vi "main.vi"() -> ()   [LabVIEW 2018]
uses:
  gbl.vi
panel:
  out "保存组数":i32
  in  "保存开关":bool
  out "监测组数":i32
  in  "监测开关":bool
  in  "采样开关":bool
  in  "报警窗":i32(listbox)
  in  "闸门四高度":i32(slide) caption="高  度" scale=0.0..50.0
  in  "闸门四宽度":i32(slide) caption="宽  度" scale=0.0..10.0
  in  "闸门四起点":i32(slide) caption="起  点" scale=0.0..10.0
  in  "闸门三高度":i32(slide) caption="高  度" scale=0.0..50.0
  in  "闸门三宽度":i32(slide) caption="宽  度" scale=0.0..10.0
  in  "闸门三起点":i32(slide) caption="起  点" scale=0.0..10.0
  in  "闸门二高度":i32(slide) caption="高  度" scale=0.0..50.0
  in  "闸门二宽度":i32(slide) caption="宽  度" scale=0.0..10.0
  in  "闸门二起点":i32(slide) caption="起  点" scale=0.0..10.0
  in  "闸门一高度":i32(slide) caption="高  度" scale=0.0..50.0
  in  "闸门一宽度":i32(slide) caption="宽  度" scale=0.0..10.0
  in  "闸门一起点":i32(slide) caption="起  点" scale=0.0..10.0
  in  "衰减上限":dbl
  in  "衰减实时值":dbl
  out "衰  减":bool
  in  "数据导出路径":string
  in  "衰减下限":dbl
  in  "声速上限":dbl
  in  "声速实时值":dbl
  out "声  速":bool
  out "连接状态":bool
  in  "本次监测名称":string
  out "实时信号":cluster{"波形数据":dbl[], "波形数据":dbl[]}[](graph)
  in  "声速下限":dbl
  in  "测    试":bool
  in  "监    测":bool
  in  "采    样":bool
  out "实时监测":cluster{"Value":timestamp[], "Value":dbl[]}[](graph)
  # "声速"
  # "衰减"
  # "时间"
  # "时间"
  # "上    限"
  # "实时值"
  # "下    限"
  # "原 始 信 号"
  # "幅值"
  # "闸  门  一"
  # "闸  门  二"
  # "闸  门  三"
  # "闸  门  四"
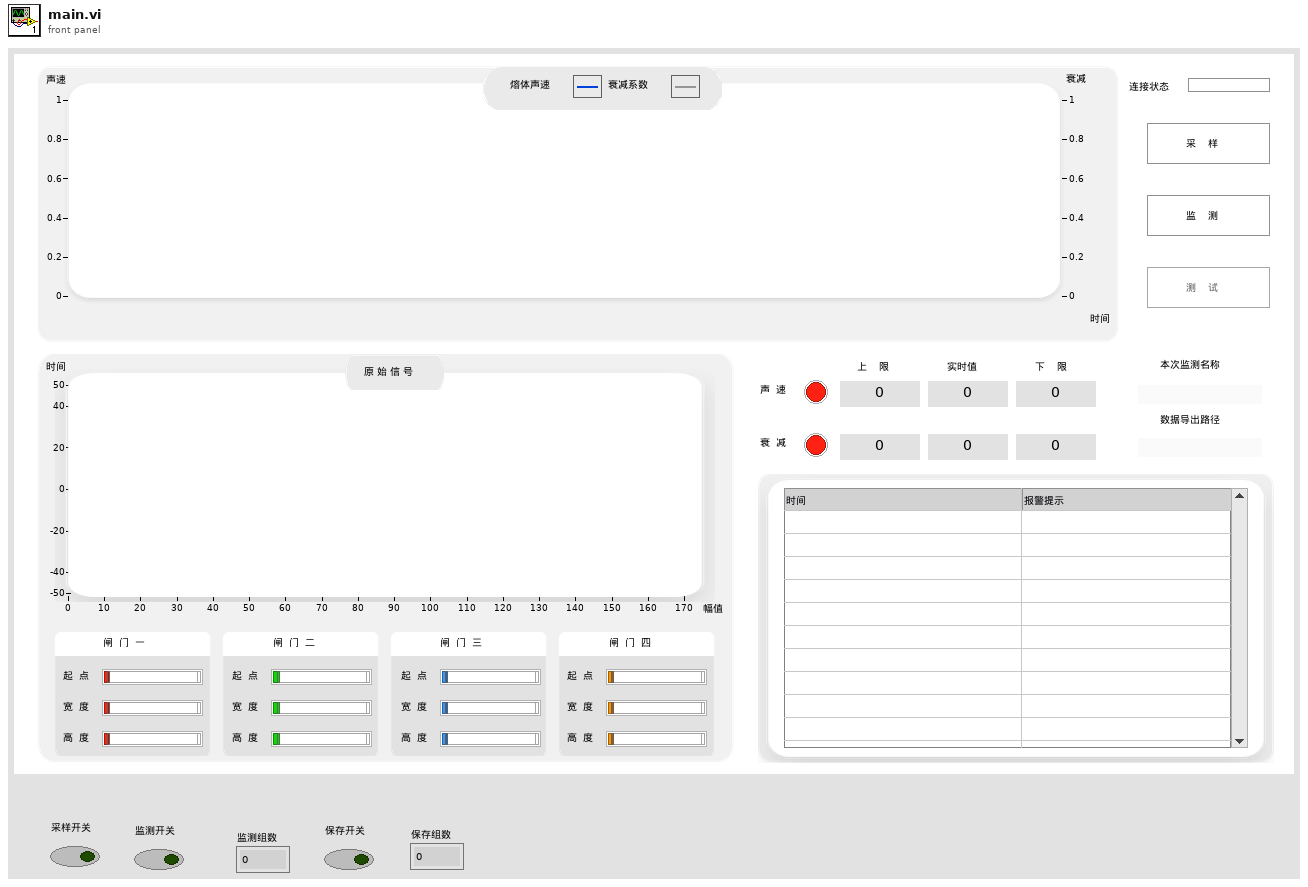
[diagram p1: front panel]
types:
  T1 = enum8{"Enabled", "Disabled", "Disabled and Grayed Out"}
  T2 = enum32{"Bad", "Idle", "Run top level", "Running"}
  T3 = enum32{"Invalid", "Standard", "Closed", "Hidden", "Minimized", "Maximized"}
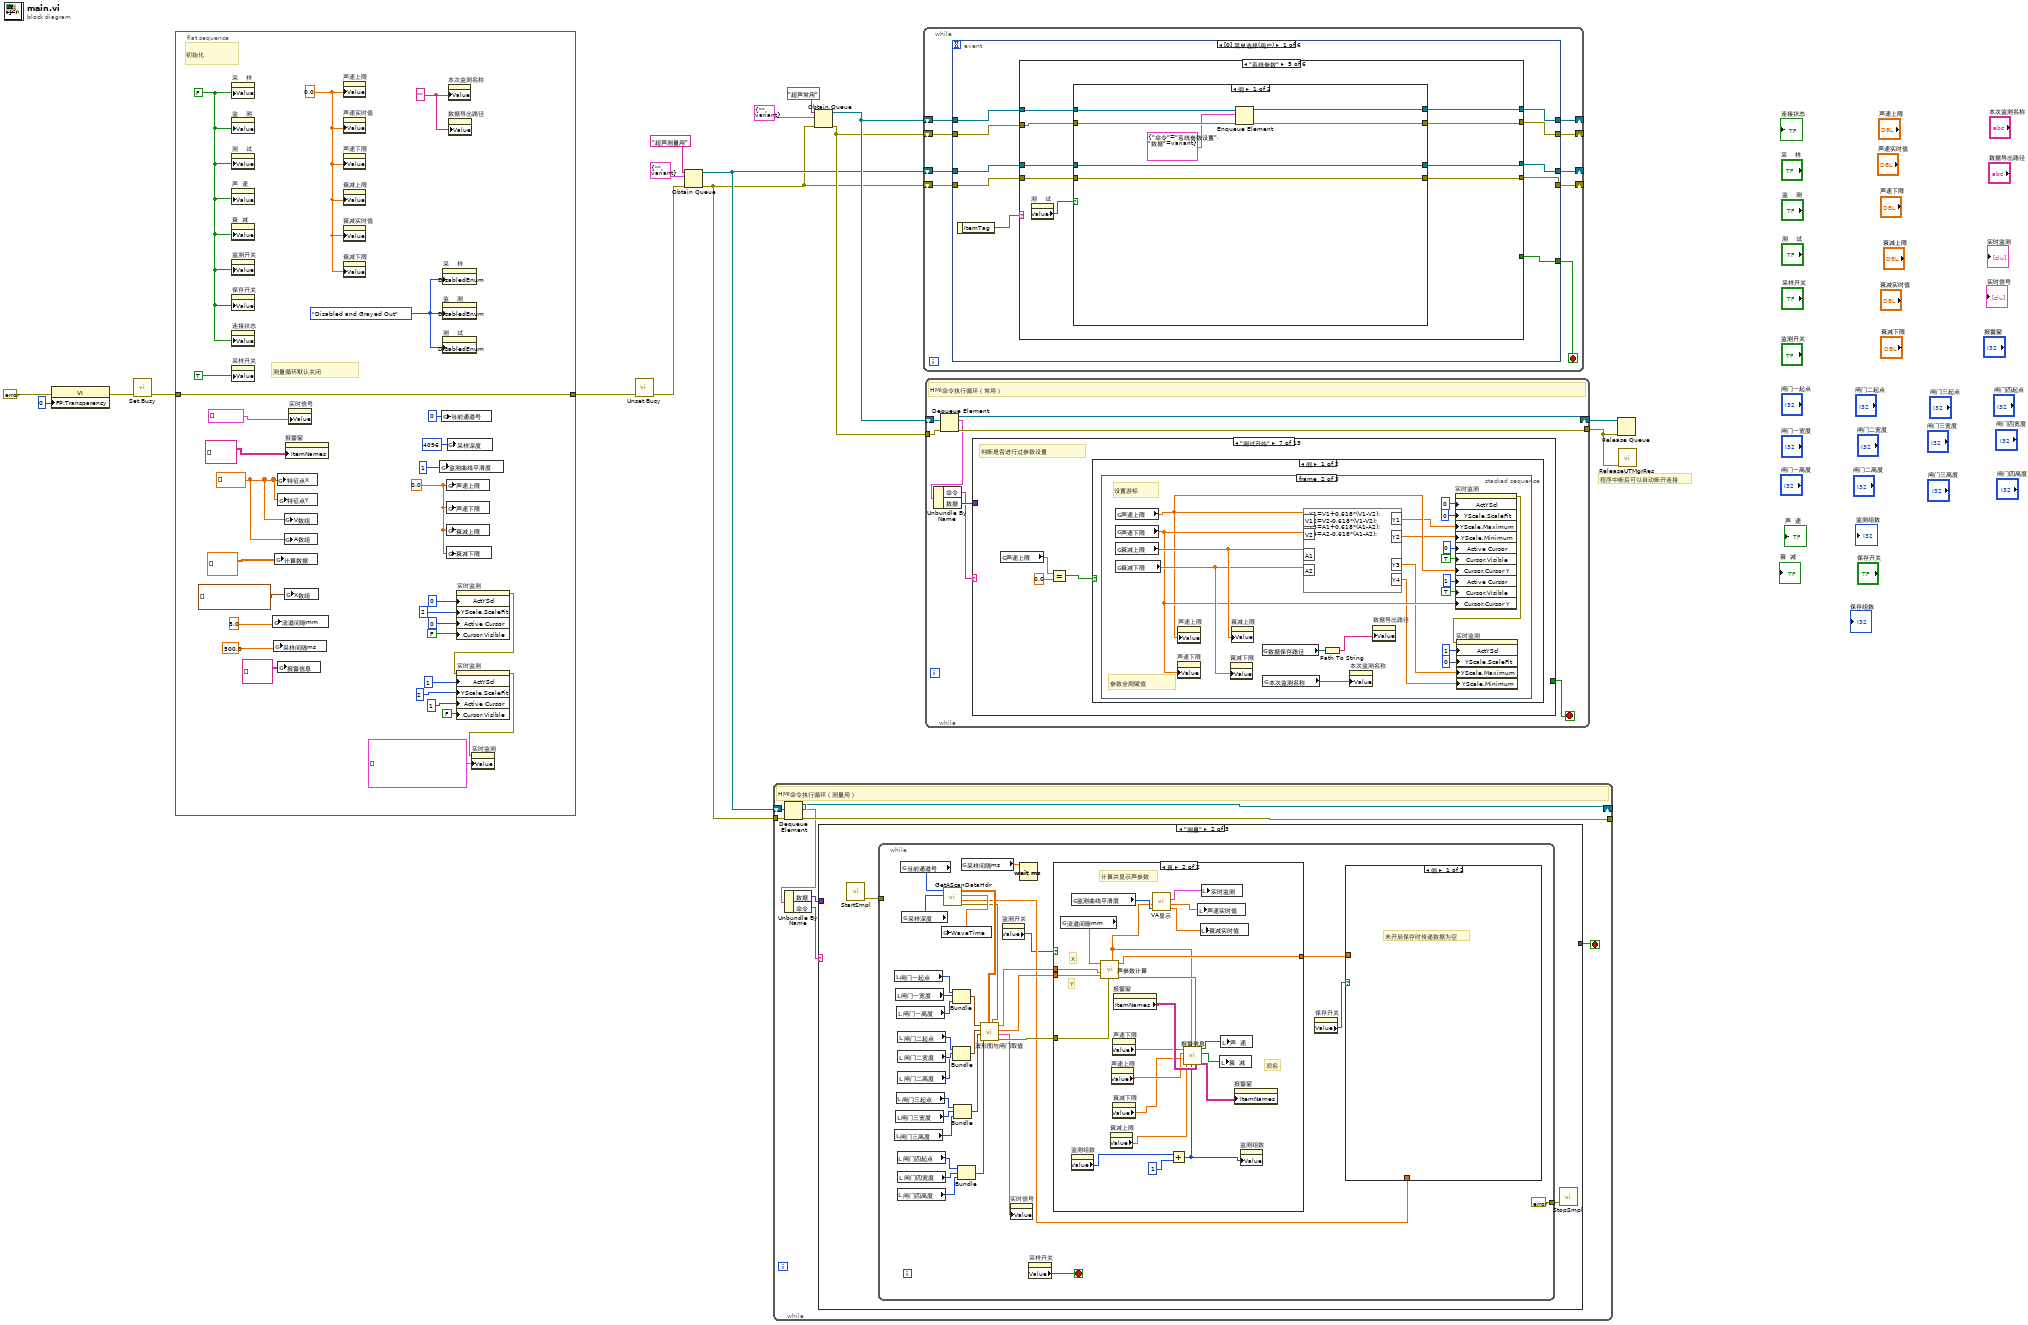
[diagram p0: block diagram]
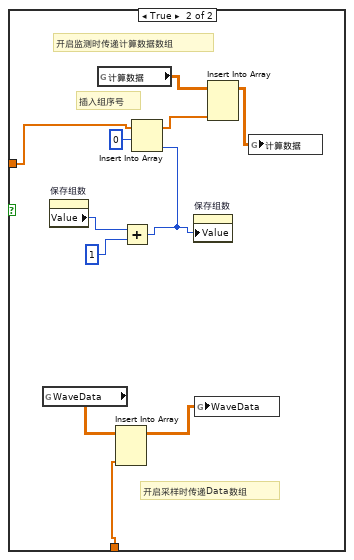
[diagram p3: hidden frame]
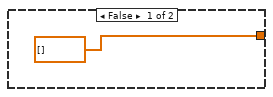
[diagram p4: hidden frame]
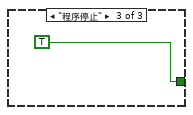
[diagram p5: hidden frame]
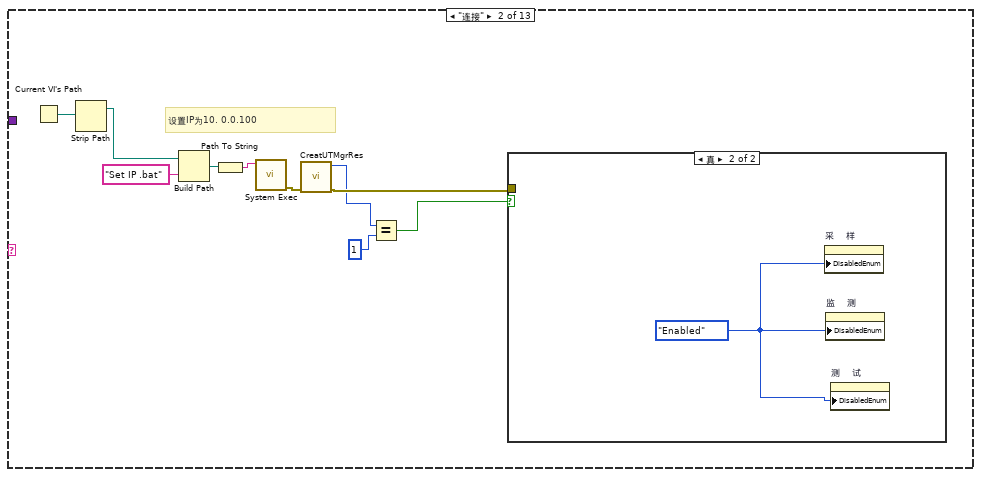
[diagram p7: hidden frame]
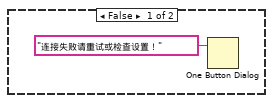
[diagram p8: hidden frame]
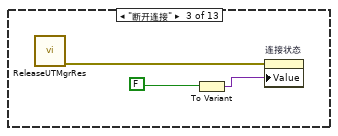
[diagram p9: hidden frame]
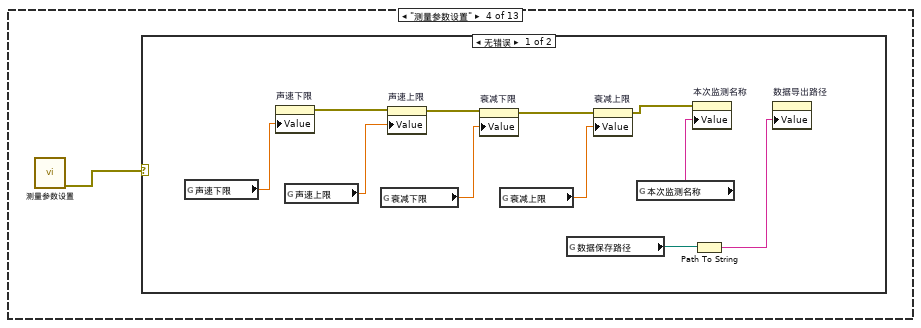
[diagram p10: hidden frame]
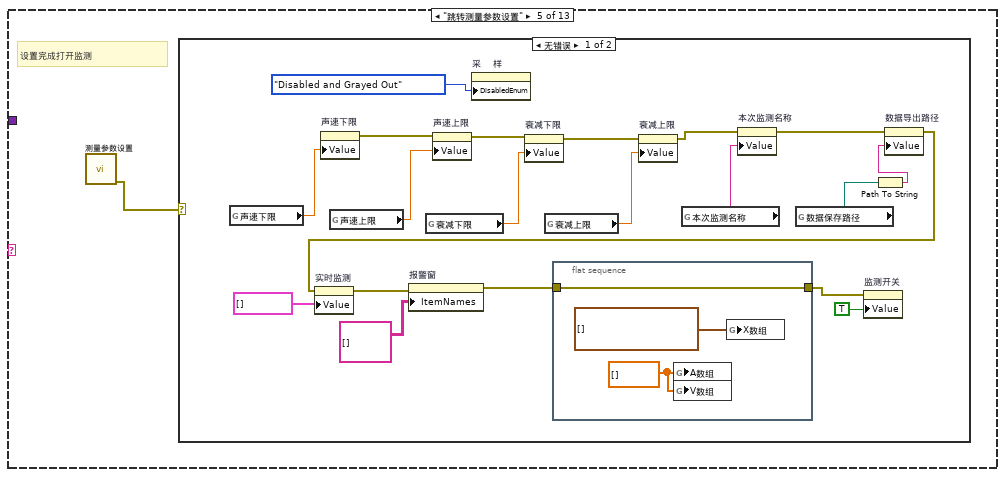
[diagram p12: hidden frame]
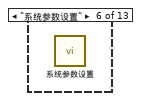
[diagram p14: hidden frame]
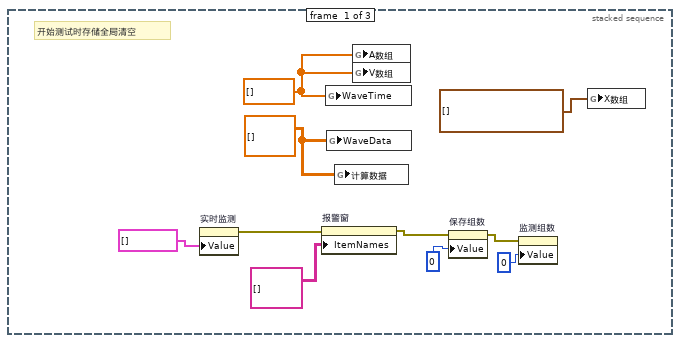
[diagram p15: hidden frame]
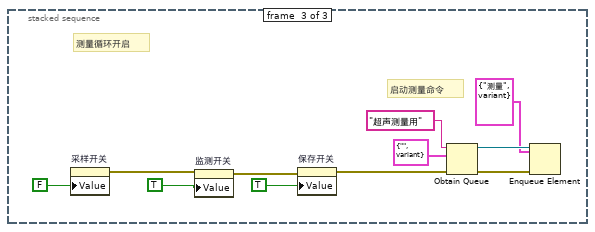
[diagram p16: hidden frame]
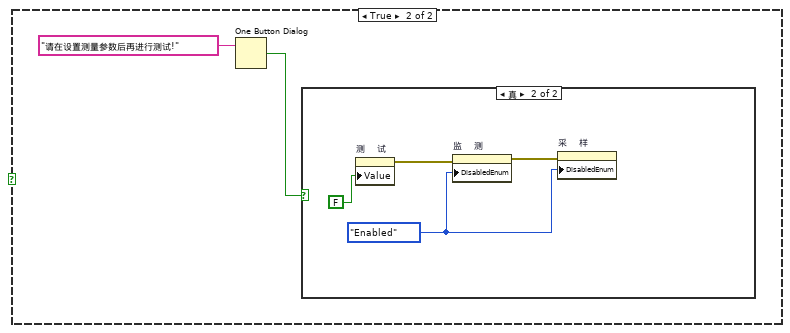
[diagram p17: hidden frame]
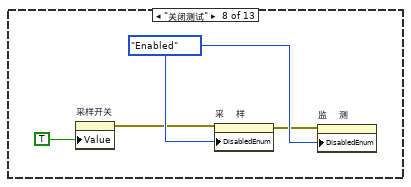
[diagram p19: hidden frame]
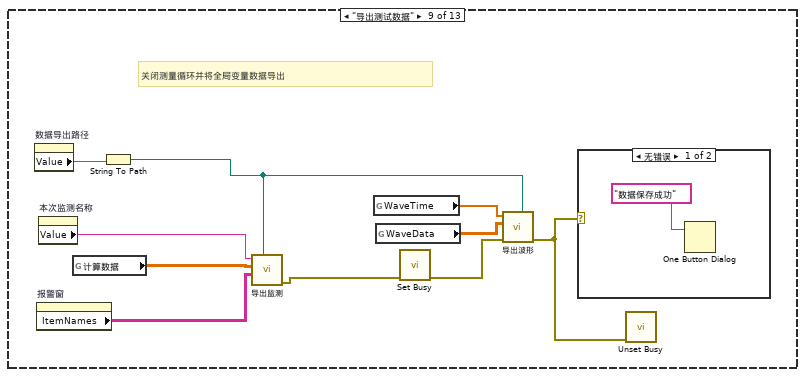
[diagram p20: hidden frame]
diagram:
  # "程序中断后可以自动断开连接"
  n1 = property class="VI"(error in=errorcluster {"status"=FALSE, "code"=0, "source"=""} ("错误输入（无错误）"), "FP:Transparency"=u8 0 ("前面板窗口:透明度")) -> (error out=w3:errorcluster)  [unwired: 1 in, 1 out]
  n2 = call <vilib>:"Set Busy.vi"("error in (no error)"=w3) -> ("error out"=w2:errorcluster)  [unwired: 9 in, 1 out]
  n3 = flat-sequence {
    tunnel: w2 -> [w35]
    tunnel: [w35] -> w1
    frame #0 {
      w41 = 0.0
      w30 = T1."Disabled and Grayed Out" ("禁用")
      w31 = ""
      w39 = dbl[] []
      w32 = 0.0
      w34 = FALSE
      # "测量循环默认关闭"
      # "初始化"
      n4 = property on="采    样" class="Bool (严格)"("Value"=w34) -> ()  [unwired: 2 in, 2 out]
      n5 = property on="监    测" class="Bool (严格)"("Value"=w34) -> ()  [unwired: 2 in, 2 out]
      n6 = property on="测    试" class="Bool (严格)"("Value"=w34) -> ()  [unwired: 2 in, 2 out]
      n7 = property on="声  速" class="Bool (严格)"("Value"=w34) -> ()  [unwired: 2 in, 2 out]
      n8 = property on="衰  减" class="Bool (严格)"("Value"=w34) -> ()  [unwired: 2 in, 2 out]
      n9 = property on="监测开关" class="Bool (严格)"("Value"=w34) -> ()  [unwired: 2 in, 2 out]
      n10 = property on="保存开关" class="Bool (严格)"("Value"=w34) -> ()  [unwired: 2 in, 2 out]
      n11 = property on="连接状态" class="Bool"("Value"=w34) -> ()  [unwired: 2 in, 2 out]
      n12 = property on="采样开关" class="Bool (严格)"("Value"=TRUE ("采样开关")) -> ()  [unwired: 2 in, 2 out]
      n13 = global write "gbl.vi" "流道间隙mm"(5.0) -> ()
      n14 = global write "gbl.vi" "采样间隔ms"(500.0) -> ()
      n15 = global write "gbl.vi" "计算数据"(dbl[][] []) -> ()
      n16 = global write "gbl.vi" "特征点X"(w39) -> ()
      n17 = global write "gbl.vi" "特征点Y"(w39) -> ()
      n18 = global write "gbl.vi" "报警信息"(string[][] [] ("报警信息")) -> ()
      n19 = global write "gbl.vi" "V数组"(w39) -> ()
      n20 = global write "gbl.vi" "A数组"(w39) -> ()
      n21 = global write "gbl.vi" "X数组"(timestamp[] []) -> ()
      n22 = property on="报警窗" class="MCListbox (严格)"("ItemNames"=string[][] []) -> ()  [unwired: 2 in, 2 out]
      n23 = property on="实时信号" class="XYGraph (严格)"("Value"=cluster{dbl[], dbl[]}[] [] ("输出数组")) -> ()  [unwired: 2 in, 2 out]
      n24 = property on="声速上限" class="DigNum (严格)"("Value"=w32) -> ()  [unwired: 2 in, 2 out]
      n25 = property on="声速实时值" class="DigNum (严格)"("Value"=w32) -> ()  [unwired: 2 in, 2 out]
      n26 = property on="声速下限" class="DigNum (严格)"("Value"=w32) -> ()  [unwired: 2 in, 2 out]
      n27 = property on="衰减上限" class="DigNum (严格)"("Value"=w32) -> ()  [unwired: 2 in, 2 out]
      n28 = property on="衰减实时值" class="DigNum (严格)"("Value"=w32) -> ()  [unwired: 2 in, 2 out]
      n29 = property on="衰减下限" class="DigNum (严格)"("Value"=w32) -> ()  [unwired: 2 in, 2 out]
      n30 = global write "gbl.vi" "监测曲线平滑度"(1) -> ()
      n31 = global write "gbl.vi" "当前通道号"(u8 0 ("当前通道号")) -> ()
      n32 = property on="采    样" class="Bool (严格)"("DisabledEnum"=w30) -> ()  [unwired: 2 in, 2 out]
      n33 = property on="监    测" class="Bool (严格)"("DisabledEnum"=w30) -> ()  [unwired: 2 in, 2 out]
      n34 = property on="测    试" class="Bool (严格)"("DisabledEnum"=w30) -> ()  [unwired: 2 in, 2 out]
      n35 = global write "gbl.vi" "声速上限"(w41) -> ()
      n36 = global write "gbl.vi" "声速下限"(w41) -> ()
      n37 = global write "gbl.vi" "衰减上限"(w41) -> ()
      n38 = global write "gbl.vi" "衰减下限"(w41) -> ()
      n39 = global write "gbl.vi" "采样深度"(4096 ("采样深度")) -> ()
      n40 = property on="本次监测名称" class="Str"("Value"=w31) -> ()  [unwired: 2 in, 2 out]
      n41 = property on="数据导出路径" class="Str"("Value"=w31) -> ()  [unwired: 2 in, 2 out]
      n42 = property on="实时监测" class="XYGraph (严格)"("ActYScl"=0 ("活动Y标尺"), "YScale.ScaleFit"=u8 2 ("Y标尺.标尺调节"), "Active Cursor"=u32 0 ("活动游标"), "Cursor.Visible"=FALSE ("游标.可见")) -> (error out=w18:errorcluster)  [unwired: 2 in, 1 out]
      n43 = property on="实时监测" class="XYGraph (严格)"(error in=w18, "ActYScl"=1 ("活动Y标尺"), "YScale.ScaleFit"=u8 2 ("Y标尺.标尺调节"), "Active Cursor"=u32 1 ("活动游标"), "Cursor.Visible"=FALSE ("游标.可见")) -> (error out=w17:errorcluster)  [unwired: 1 in, 1 out]
      n44 = property on="实时监测" class="XYGraph (严格)"(error in=w17, "Value"=cluster{"Value":timestamp[], "Value":dbl[]}[] [] ("实时监测")) -> ()  [unwired: 1 in, 2 out]
    }
  }
  n45 = call <vilib>:"Unset Busy.vi"("error in (no error)"=w1) -> ("error out"=w16:errorcluster)  [unwired: 10 in]
  n46 = Obtain Queue(name (unnamed)="超声测量用" ("名称（未命名）"), element data type=cluster{"命令":string, "数据":variant} {"命令"="", "数据"=variant}, error in (no error)=w16) -> (queue out=w7:refnum<queue>, error out=w6:errorcluster)  [unwired: 2 in, 1 out]
  n47 = while {
    shift-right: [w52] -> _
    shift-left: w7 -> [w53]
    tunnel: [w51] -> _
    tunnel: w6 -> [w48]
    stop <- w49 stop-if-true
    # "HMI命令执行循环（测量用）"
    n48 = Dequeue Element(queue=w53, error in (no error)=w48) -> (queue out=w52:refnum<queue>, element=w47:cluster{"命令":string, "数据":variant}, error out=w51:errorcluster)  [unwired: 1 in, 1 out]
    n49 = Unbundle By Name(w47) -> ("数据"=w50:variant, "命令"=w46:string)
    n50 = case shown="\"测量\"" w46 {
      tunnel: w50 -> [_ _ _]
      tunnel: [_ _ TRUE] -> w49
      frame "空", Default {
      }
      frame "测量" {
        n51 = call "StartSmpl.vi"() -> ("错误输出"=w55:errorcluster)  [unwired: 11 in]
        n52 = while {
          tunnel: w55 -> [_]
          tunnel: [errorcluster {"status"=FALSE, "code"=0, "source"=""} ("错误输入（无错误）")] -> w54
          stop <- w74 stop-if-true
          n53 = local read "闸门一起点"() -> (w73:i32)
          n54 = local read "闸门三高度"() -> (w63:i32)
          n55 = local read "闸门一宽度"() -> (w72:i32)
          n56 = local read "闸门三宽度"() -> (w64:i32)
          n57 = local read "闸门三起点"() -> (w65:i32)
          n58 = local read "闸门一高度"() -> (w71:i32)
          n59 = local read "闸门四起点"() -> (w61:i32)
          n60 = local read "闸门四高度"() -> (w59:i32)
          n61 = local read "闸门二起点"() -> (w69:i32)
          n62 = local read "闸门二宽度"() -> (w68:i32)
          n63 = local read "闸门二高度"() -> (w67:i32)
          n64 = local read "闸门四宽度"() -> (w60:i32)
          n65 = global read "gbl.vi" "当前通道号"() -> (w81:u8)
          n66 = global read "gbl.vi" "采样深度"() -> (w80:i32)
          n67 = call "GetAScanDataHdr.vi"("采样深度"=w80, "需要获取的通道"=w81) -> ("错误输出"=w79:errorcluster, "Data"=w77:dbl[], "Time"=w84:dbl[], "波形数据"=w85:dbl[][])  [unwired: 6 in]
          n68 = global write "gbl.vi" "WaveTime"(w84) -> ()
          n69 = Bundle("闸门一起点"=w73, "闸门一宽度"=w72, "闸门一高度"=w71) -> (w70:cluster{"闸门一起点":i32, "闸门一宽度":i32, "闸门一高度":i32})  [unwired: 1 in]
          n70 = Bundle("闸门二起点"=w69, "闸门二宽度"=w68, "闸门二高度"=w67) -> (w66:cluster{"闸门二起点":i32, "闸门二宽度":i32, "闸门二高度":i32})  [unwired: 1 in]
          n71 = Bundle("闸门三起点"=w65, "闸门三宽度"=w64, "闸门三高度"=w63) -> (w62:cluster{"闸门三起点":i32, "闸门三宽度":i32, "闸门三高度":i32})  [unwired: 1 in]
          n72 = Bundle("闸门四起点"=w61, "闸门四宽度"=w60, "闸门四高度"=w59) -> (w58:cluster{"闸门四起点":i32, "闸门四宽度":i32, "闸门四高度":i32})  [unwired: 1 in]
          n73 = global read "gbl.vi" "采样间隔ms"() -> (w82:dbl)
          n74 = call "波形图与闸门取值.vi"("错误输入"=w79, "波形数据"=w85, "闸门 4"=w58, "闸门 3"=w62, "闸门 2"=w66, "闸门"=w70) -> ("错误输出"=w78:errorcluster, "XY图"=w57:cluster{"波形数据":dbl[], "波形数据":dbl[]}[], "Y"=w86:dbl[], "X"=w87:dbl[])  [unwired: 2 in]
          n75 = property on="监测开关" class="Bool (严格)"() -> ("Value"=w75:bool)  [unwired: 2 in, 2 out]
          n76 = property on="实时信号" class="XYGraph (严格)"("Value"=w57) -> ()  [unwired: 2 in, 2 out]
          n77 = Wait (ms)(milliseconds to wait=w82) -> ()  [unwired: 1 out]
          n78 = property on="采样开关" class="Bool (严格)"() -> ("Value"=w74:bool)  [unwired: 2 in, 2 out]
          n79 = case shown="真" w75 {
            tunnel: w87 -> [_ w121]
            tunnel: w86 -> [_ w120]
            tunnel: [dbl[] [] w116] -> w83
            tunnel: w78 -> [_ w119]
            frame False {
            }
            frame True {
              # "项名"
              # "计算并显示声参数"
              # "Y"
              # "X"
              n80 = global read "gbl.vi" "流道间隙mm"() -> (w113:dbl)
              n81 = global read "gbl.vi" "监测曲线平滑度"() -> (w117:i32)
              n82 = property on="监测组数" class="DigNum (严格)"() -> ("Value"=w101:i32)  [unwired: 2 in, 2 out]
              n83 = call "声参数计算.vi"("错误输入"=w119, "Y"=w120, "X"=w121, "流道间隙"=w113) -> ("错误输出"=w115:errorcluster, "计算数据"=w116:dbl[], "声参数"=w114:dbl[])  [unwired: 4 in]
              n84 = property on="衰减上限" class="DigNum (严格)"() -> ("Value"=w105:dbl)  [unwired: 2 in, 2 out]
              n85 = property on="声速上限" class="DigNum (严格)"() -> ("Value"=w107:dbl)  [unwired: 2 in, 2 out]
              n86 = property on="声速下限" class="DigNum (严格)"() -> ("Value"=w108:dbl)  [unwired: 2 in, 2 out]
              n87 = property on="衰减下限" class="DigNum (严格)"() -> ("Value"=w106:dbl)  [unwired: 2 in, 2 out]
              n88 = property on="报警窗" class="MCListbox (严格)"() -> ("ItemNames"=w109:string[][])  [unwired: 2 in, 2 out]
              n89 = call "VA显示.vi"("平滑程度"=w117, "声参数"=w114) -> ("实时A"=w110:dbl, "实时V"=w111:dbl, "XY图"=w112:cluster{"Value":timestamp[], "Value":dbl[]}[])  [unwired: 4 in]
              n90 = Add(x=w101, y=1) -> (x+y=w100:i32)
              n91 = call "报警信息.vi"("报警信息输入"=w109, "错误输入"=w115, "当前组"=w100, "声参数"=w114, "衰减上限"=w105, "衰减下限"=w106, "声速上限"=w107, "声速下限"=w108) -> ("报警信息输出"=w104:string[][], "衰减"=w103:bool, "声速"=w102:bool)  [unwired: 1 out]
              n92 = local write "声速实时值"(w111) -> ()
              n93 = local write "衰减实时值"(w110) -> ()
              n94 = local write "实时监测"(w112) -> ()
              n95 = local write "衰  减"(w103) -> ()
              n96 = local write "声  速"(w102) -> ()
              n97 = property on="报警窗" class="MCListbox (严格)"("ItemNames"=w104) -> ()  [unwired: 2 in, 2 out]
              n98 = property on="监测组数" class="DigNum (严格)"("Value"=w100) -> ()  [unwired: 2 in, 2 out]
            }
          }
          n99 = property on="保存开关" class="Bool (严格)"() -> ("Value"=w56:bool)  [unwired: 2 in, 2 out]
          n100 = case shown="假" w56 {
            tunnel: w77 -> [_ w98]
            tunnel: w83 -> [_ w90]
            frame False {
              # "未开启保存时传递数据为空"
            }
            frame True {
              # "插入组序号"
              # "开启监测时传递计算数据数组"
              # "开启采样时传递Data数组"
              n101 = global read "gbl.vi" "WaveData"() -> (w95:dbl[][])
              n102 = property on="保存组数" class="DigNum (严格)"() -> ("Value"=w89:i32)  [unwired: 2 in, 2 out]
              n103 = global read "gbl.vi" "计算数据"() -> (w92:dbl[][])
              n104 = Insert Into Array(array=w95, new element=w98) -> (w94:dbl[][])  [unwired: 2 in]
              n105 = Add(x=w89, y=1) -> (x+y=w88:i32)
              n106 = Insert Into Array(array=w90, index=0 ("索引"), new element=w88) -> (w97:dbl[])
              n107 = property on="保存组数" class="DigNum (严格)"("Value"=w88) -> ()  [unwired: 2 in, 2 out]
              n108 = global write "gbl.vi" "WaveData"(w94) -> ()
              n109 = Insert Into Array(array=w92, new element=w97) -> (w93:dbl[][])  [unwired: 2 in]
              n110 = global write "gbl.vi" "计算数据"(w93) -> ()
            }
          }
        }
        n111 = call "StopSmpl.vi"("错误输入（无错误）"=w54) -> ()  [unwired: 10 in, 1 out]
      }
      frame "程序停止" {
      }
    }
  }
  n112 = Obtain Queue(name (unnamed)="超声常用" ("名称（未命名）"), element data type=cluster{"命令":string, "数据":variant} {"命令"="", "数据"=variant}, error in (no error)=w6) -> (queue out=w12:refnum<queue>, error out=w11:errorcluster)  [unwired: 2 in, 1 out]
  n113 = while {
    shift-right: [w129] -> _
    shift-left: w6 -> [w130]
    shift-right: [w127] -> _
    shift-left: w7 -> [w131]
    shift-right: [w123] -> _
    shift-left: w12 -> [w126]
    shift-right: [w124] -> _
    shift-left: w11 -> [w125]
    stop <- w128 stop-if-true
    n114 = event shown="[0] 菜单选择(用户)" {
      selector: _ -> [_ _ _ _ _ _]
      dyn-events: _ -> [_ _ _ _ _ _]
      timeout: _ -> [_ _ _ _ _ _]
      tunnel: w131 -> [w140 w256 w279 w349 w371 w385]
      tunnel: w130 -> [w138 w253 w277 w347 w370 w384]
      tunnel: [w137 w254 w276 w346 w370 w383] -> w129
      tunnel: [w136 _ _ _ _ w379] -> w128
      tunnel: [w139 w255 w278 w348 w371 w382] -> w127
      tunnel: w126 -> [w135 w252 w275 w345 w369 w387]
      tunnel: w125 -> [w134 w251 w274 w343 w367 w386]
      tunnel: [w133 w249 w272 w342 w366 w381] -> w124
      tunnel: [w132 w250 w273 w344 w368 w380] -> w123
      event Menu Selection (User) {
        n115 = event-data() -> ("ItemTag"=w141:string)  [unwired: 1 in]
        n116 = case shown="\"系统参数\"" w141 {
          tunnel: w140 -> [w147 w157 w180 w207 w224 w242]
          tunnel: [w147 w156 w179 w206 w222 w242] -> w139
          tunnel: w138 -> [w148 w155 w177 w204 w223 w241]
          tunnel: [w148 w154 w178 w205 w221 w241] -> w137
          tunnel: [_ _ w176 _ _ _] -> w136
          tunnel: w135 -> [w146 w153 w175 w203 w228 w247]
          tunnel: w134 -> [w144 w151 w174 w202 w226 w245]
          tunnel: [w143 w150 w172 w200 w225 w244] -> w133
          tunnel: [w142 w152 w173 w201 w227 w246] -> w132
          frame "连接", Default {
            n117 = Enqueue Element(queue=w146, element=cluster{"命令":string, "数据":variant} {"命令"="连接", "数据"=variant} ("元素"), error in (no error)=w144) -> (queue out=w142:refnum<queue>, error out=w143:errorcluster)  [unwired: 1 in, 1 out]
          }
          frame "断开连接" {
            n118 = property on="采    样" class="Bool (严格)"() -> ("Value"=w149:bool)  [unwired: 2 in, 2 out]
            n119 = case shown="假" w149 {
              tunnel: w157 -> [w164 w169]
              tunnel: [w164 w169] -> w156
              tunnel: w155 -> [w163 w168]
              tunnel: [w163 w168] -> w154
              tunnel: [w158 w166] -> w152
              tunnel: w153 -> [w160 w166]
              tunnel: [w161 w165] -> w150
              tunnel: w151 -> [w162 w165]
              frame False {
                n120 = Enqueue Element(queue=w160, element=cluster{"命令":string, "数据":variant} {"命令"="断开连接", "数据"=variant} ("元素"), error in (no error)=w162) -> (queue out=w158:refnum<queue>, error out=w161:errorcluster)  [unwired: 1 in, 1 out]
              }
              frame True {
                n121 = One Button Dialog(message="请先关闭采样！" ("消息")) -> ()  [unwired: 1 in, 1 out]
              }
            }
          }
          frame "退出软件" {
            n122 = Two Button Dialog(message="是否退出超声软件？" ("消息")) -> (T button?=w170:bool)  [unwired: 2 in]
            n123 = case shown="真" w170 {
              tunnel: [FALSE TRUE] -> w176
              tunnel: w175 -> [w184 w197]
              tunnel: [w184 w196] -> w173
              tunnel: w174 -> [w183 w188]
              tunnel: [w183 w195] -> w172
              tunnel: [w182 w193] -> w179
              tunnel: w180 -> [w182 w194]
              tunnel: [w181 w191] -> w178
              tunnel: w177 -> [w181 w192]
              frame False {
              }
              frame True {
                w190 = cluster{"命令":string, "数据":variant} {"命令"="程序停止", "数据"=variant} ("元素")
                n124 = Enqueue Element(queue=w197, element=cluster{"命令":string, "数据":variant} {"命令"="关闭测试", "数据"=variant} ("元素"), error in (no error)=w188) -> (queue out=w189:refnum<queue>, error out=w187:errorcluster)  [unwired: 1 in, 1 out]
                n125 = Enqueue Element(queue=w189, element=w190, error in (no error)=w187) -> (queue out=w196:refnum<queue>, error out=w195:errorcluster)  [unwired: 1 in, 1 out]
                n126 = Enqueue Element(queue=w194, element=w190, error in (no error)=w192) -> (queue out=w193:refnum<queue>, error out=w191:errorcluster)  [unwired: 1 in, 1 out]
              }
            }
          }
          frame "测量参数" {
            n127 = property on="测    试" class="Bool (严格)"() -> ("Value"=w199:bool)  [unwired: 2 in, 2 out]
            n128 = case shown="假" w199 {
              tunnel: w207 -> [w211 w214]
              tunnel: [w211 w214] -> w206
              tunnel: [w210 w213] -> w205
              tunnel: w204 -> [w210 w213]
              tunnel: [w209 w218] -> w201
              tunnel: w203 -> [w209 w219]
              tunnel: [w208 w216] -> w200
              tunnel: w202 -> [w208 w217]
              frame True {
                n129 = One Button Dialog(message="测量时不能进行测量参数设置！" ("消息")) -> ()  [unwired: 1 in, 1 out]
              }
              frame False {
                n130 = Enqueue Element(queue=w219, element=cluster{"命令":string, "数据":variant} {"命令"="测量参数设置", "数据"=variant} ("元素"), error in (no error)=w217) -> (queue out=w218:refnum<queue>, error out=w216:errorcluster)  [unwired: 1 in, 1 out]
              }
            }
          }
          frame "系统参数" {
            n131 = property on="测    试" class="Bool (严格)"() -> ("Value"=w220:bool)  [unwired: 2 in, 2 out]
            n132 = case shown="假" w220 {
              tunnel: w228 -> [w235 w239]
              tunnel: [w234 w239] -> w227
              tunnel: w226 -> [w233 w238]
              tunnel: [w232 w238] -> w225
              tunnel: w224 -> [w230 w237]
              tunnel: w223 -> [w229 w236]
              tunnel: [w230 w237] -> w222
              tunnel: [w229 w236] -> w221
              frame False {
                n133 = Enqueue Element(queue=w235, element=cluster{"命令":string, "数据":variant} {"命令"="系统参数设置", "数据"=variant} ("元素"), error in (no error)=w233) -> (queue out=w234:refnum<queue>, error out=w232:errorcluster)  [unwired: 1 in, 1 out]
              }
              frame True {
                n134 = One Button Dialog(message="保存过程中不能进行系统参数设置" ("消息")) -> ()  [unwired: 1 in, 1 out]
              }
            }
          }
          frame "导出数据" {
            n135 = Enqueue Element(queue=w247, element=cluster{"命令":string, "数据":variant} {"命令"="导出测试数据", "数据"=variant} ("元素"), error in (no error)=w245) -> (queue out=w246:refnum<queue>, error out=w244:errorcluster)  [unwired: 1 in, 1 out]
          }
        }
      }
      event "采    样": Value Change {
        n136 = event-data() -> ("NewVal"=w248:bool)  [unwired: 1 in, 5 out]
        n137 = case shown="真" w248 {
          tunnel: w256 -> [w266 w269]
          tunnel: [w265 w269] -> w255
          tunnel: [w264 w270] -> w254
          tunnel: w253 -> [w263 w270]
          tunnel: [w261 w268] -> w250
          tunnel: w252 -> [w261 w268]
          tunnel: [w260 w267] -> w249
          tunnel: w251 -> [w260 w267]
          frame True {
            # "开启测量循环"
            # "开启采样"
            n138 = property on="采样开关" class="Bool (严格)"("Value"=FALSE ("采样开关")) -> (error out=w259:errorcluster)  [unwired: 2 in, 1 out]
            n139 = Enqueue Element(queue=w266, element=cluster{"命令":string, "数据":variant} {"命令"="测量", "数据"=variant} ("元素"), error in (no error)=w263) -> (queue out=w265:refnum<queue>, error out=w264:errorcluster)  [unwired: 1 in, 1 out]
            n140 = property on="监    测" class="Bool (严格)"(error in=w259, "DisabledEnum"=T1."Enabled" ("禁用")) -> ()  [unwired: 1 in, 2 out]
          }
          frame False {
            # "关闭采样"
          }
        }
      }
      event "监    测": Value Change {
        # "开启监测时时禁用采样，恢复保存，并弹窗输入参数"
        n141 = event-data() -> ("NewVal"=w271:bool)  [unwired: 1 in, 5 out]
        n142 = case shown="真" w271 {
          tunnel: w279 -> [w285 w294]
          tunnel: [w285 w291] -> w278
          tunnel: w277 -> [w286 w293]
          tunnel: [w286 w292] -> w276
          tunnel: [w284 w289] -> w273
          tunnel: w275 -> [w284 w290]
          tunnel: [w283 w287] -> w272
          tunnel: w274 -> [w283 w288]
          frame False {
            n143 = property on="监测开关" class="Bool (严格)"("Value"=FALSE) -> (error out=w280:errorcluster)  [unwired: 2 in, 1 out]
            n144 = property on="采    样" class="Bool (严格)"(error in=w280, "DisabledEnum"=T1."Enabled" ("禁用")) -> ()  [unwired: 1 in, 2 out]
          }
          frame True {
            # "判断是否进行过\n测量参数设置"
            n145 = global read "gbl.vi" "声速上限"() -> (w297:dbl)
            n146 = Equal?(x=w297, y=0.0) -> (x = y?=w295:bool)
            n147 = case shown="真" w295 {
              tunnel: [w330 w335] -> w291
              tunnel: w294 -> [w330 w335]
              tunnel: [w329 w334] -> w292
              tunnel: w293 -> [w329 w334]
              tunnel: w290 -> [w328 w340]
              tunnel: [w328 w339] -> w289
              tunnel: [w327 w337] -> w287
              tunnel: w288 -> [w327 w338]
              frame False {
                n148 = global read "gbl.vi" "声速下限"() -> (w317:dbl)
                n149 = property on="声速下限" class="DigNum (严格)"("Value"=w317) -> (error out=w321:errorcluster)  [unwired: 2 in, 1 out]
                n150 = global read "gbl.vi" "声速上限"() -> (w320:dbl)
                n151 = property on="采    样" class="Bool (严格)"("DisabledEnum"=T1."Disabled and Grayed Out" ("禁用")) -> ()  [unwired: 2 in, 2 out]
                n152 = global read "gbl.vi" "衰减下限"() -> (w318:dbl)
                n153 = property on="声速上限" class="DigNum (严格)"(error in=w321, "Value"=w320) -> (error out=w323:errorcluster)  [unwired: 1 in, 1 out]
                n154 = property on="衰减下限" class="DigNum (严格)"(error in=w323, "Value"=w318) -> (error out=w324:errorcluster)  [unwired: 1 in, 1 out]
                n155 = global read "gbl.vi" "衰减上限"() -> (w322:dbl)
                n156 = flat-sequence {
                  tunnel: [w331] -> w299
                  tunnel: w300 -> [w331]
                  frame #0 {
                    w332 = dbl[] []
                    n157 = global write "gbl.vi" "X数组"(timestamp[] []) -> ()
                    n158 = global write "gbl.vi" "A数组"(w332) -> ()
                    n159 = global write "gbl.vi" "V数组"(w332) -> ()
                  }
                }
                n160 = property on="衰减上限" class="DigNum (严格)"(error in=w324, "Value"=w322) -> (error out=w325:errorcluster)  [unwired: 1 in, 1 out]
                n161 = global read "gbl.vi" "本次监测名称"() -> (w319:string)
                n162 = property on="本次监测名称" class="Str"(error in=w325, "Value"=w319) -> (error out=w312:errorcluster)  [unwired: 1 in, 1 out]
                n163 = property on="实时监测" class="XYGraph (严格)"(error in=w312, "ActYScl"=0 ("活动Y标尺"), "YScale.ScaleFit"=u8 2 ("Y标尺.标尺调节"), "Active Cursor"=u32 0 ("活动游标"), "Cursor.Visible"=FALSE ("游标.可见")) -> (error out=w298:errorcluster)  [unwired: 1 in, 1 out]
                n164 = property on="实时监测" class="XYGraph (严格)"(error in=w298, "ActYScl"=1 ("活动Y标尺"), "YScale.ScaleFit"=u8 2 ("Y标尺.标尺调节"), "Active Cursor"=u32 1 ("活动游标"), "Cursor.Visible"=FALSE ("游标.可见")) -> (error out=w306:errorcluster)  [unwired: 1 in, 1 out]
                n165 = property on="实时监测" class="XYGraph (严格)"(error in=w306, "Value"=cluster{"数组":timestamp[], dbl[]}[] [] ("实时监测")) -> (error out=w305:errorcluster)  [unwired: 1 in, 1 out]
                n166 = property on="报警窗" class="MCListbox (严格)"(error in=w305, "ItemNames"=string[][] []) -> (error out=w302:errorcluster)  [unwired: 1 in, 1 out]
                n167 = property on="监测组数" class="DigNum (严格)"(error in=w302, "Value"=0 ("监测组数")) -> (error out=w300:errorcluster)  [unwired: 1 in, 1 out]
                n168 = property on="监测开关" class="Bool (严格)"(error in=w299, "Value"=TRUE) -> ()  [unwired: 1 in, 2 out]
              }
              frame True {
                n169 = Enqueue Element(queue=w340, element=cluster{"命令":string, "数据":variant} {"命令"="跳转测量参数设置", "数据"=variant} ("元素"), error in (no error)=w338) -> (queue out=w339:refnum<queue>, error out=w337:errorcluster)  [unwired: 1 in, 1 out]
              }
            }
          }
        }
      }
      event "测    试": Value Change {
        n170 = event-data() -> ("NewVal"=w341:bool)  [unwired: 1 in, 5 out]
        n171 = case shown="真" w341 {
          tunnel: w349 -> [w351 w358]
          tunnel: [w351 w358] -> w348
          tunnel: w347 -> [w350 w357]
          tunnel: [w350 w357] -> w346
          tunnel: w345 -> [w356 w359]
          tunnel: [w355 w363] -> w344
          tunnel: w343 -> [w354 w362]
          tunnel: [w353 w361] -> w342
          frame False {
            n172 = Enqueue Element(queue=w356, element=cluster{"命令":string, "数据":variant} {"命令"="关闭测试", "数据"=variant} ("元素"), error in (no error)=w354) -> (queue out=w355:refnum<queue>, error out=w353:errorcluster)  [unwired: 1 in, 1 out]
          }
          frame True {
            n173 = Enqueue Element(queue=w359, element=cluster{"命令":string, "数据":variant} {"命令"="测试开始", "数据"=variant} ("元素"), error in (no error)=w362) -> (queue out=w363:refnum<queue>, error out=w361:errorcluster)  [unwired: 1 in, 1 out]
          }
        }
      }
      event "实时监测": Mouse Down {
        n174 = event-data() -> ("Mods"=w365:cluster{"Double Click":bool, "Menu Key":bool})  [unwired: 1 in, 7 out]
        n175 = Unbundle By Name(w365) -> ("Double Click"=w364:bool)
        n176 = case shown="真" w364 {
          tunnel: w369 -> [w373 w378]
          tunnel: [w373 w377] -> w368
          tunnel: w367 -> [w372 w376]
          tunnel: [w372 w375] -> w366
          frame False {
          }
          frame True {
            n177 = Enqueue Element(queue=w378, element=cluster{"命令":string, "数据":variant} {"命令"="放大实时监测图", "数据"=variant} ("元素"), error in (no error)=w376) -> (queue out=w377:refnum<queue>, error out=w375:errorcluster)  [unwired: 1 in, 1 out]
          }
        }
      }
      event Panel Close? {
        n178 = event-data() -> ()  [unwired: 1 in, 1 out]
        n179 = Current VI's Path() -> (path=w388:path)
        n180 = Strip Path(path=w388) -> (stripped path=w389:path)  [unwired: 1 out]
        n181 = Strip Path(path=w389) -> (stripped path=w390:path)  [unwired: 1 out]
        n182 = Build Path(base path=w390, name or relative path="主程序界面.vi" ("名称或相对路径")) -> (appended path=w392:path)
        n183 = Open VI Reference(vi path=w392) -> (vi reference=w393:refnum<vi>)  [unwired: 5 in, 1 out]
        n184 = property class="VI"(reference=w393) -> ("Exec.State"=w394:T2)  [unwired: 1 in, 2 out]
        n185 = case shown="\"Bad\", 默认" w394 {
          tunnel: w387 -> [w402 w428]
          tunnel: w386 -> [w401 w426]
          tunnel: w385 -> [w404 w430]
          tunnel: w384 -> [w403 w429]
          tunnel: [w398 w430] -> w382
          tunnel: [w397 w429] -> w383
          tunnel: [w400 w427] -> w380
          tunnel: [w399 w425] -> w381
          tunnel: [w396 _] -> w379
          frame "Bad", Default {
            n186 = Two Button Dialog(message="是否退出超声软件？" ("消息")) -> (T button?=w405:bool)  [unwired: 2 in]
            n187 = case shown="真" w405 {
              tunnel: w404 -> [w408 w422]
              tunnel: w403 -> [w407 w418]
              tunnel: w402 -> [w410 w423]
              tunnel: w401 -> [w409 w413]
              tunnel: [w410 w421] -> w400
              tunnel: [w409 w419] -> w399
              tunnel: [w408 w420] -> w398
              tunnel: [w407 w417] -> w397
              tunnel: [_ TRUE] -> w396
              frame False {
              }
              frame True {
                w416 = cluster{"命令":string, "数据":variant} {"命令"="程序停止", "数据"=variant} ("元素")
                n188 = Enqueue Element(queue=w423, element=cluster{"命令":string, "数据":variant} {"命令"="关闭测试", "数据"=variant} ("元素"), error in (no error)=w413) -> (queue out=w414:refnum<queue>, error out=w412:errorcluster)  [unwired: 1 in, 1 out]
                n189 = Enqueue Element(queue=w414, element=w416, error in (no error)=w412) -> (queue out=w421:refnum<queue>, error out=w419:errorcluster)  [unwired: 1 in, 1 out]
                n190 = Enqueue Element(queue=w422, element=w416, error in (no error)=w418) -> (queue out=w420:refnum<queue>, error out=w417:errorcluster)  [unwired: 1 in, 1 out]
              }
            }
          }
          frame "Run top level" {
            n191 = Enqueue Element(queue=w428, element=cluster{"命令":string, "数据":variant} {"命令"="前面板消失", "数据"=variant} ("元素"), error in (no error)=w426) -> (queue out=w427:refnum<queue>, error out=w425:errorcluster)  [unwired: 1 in, 1 out]
          }
        }
        n192 = event-data("Discard?"=TRUE ("放弃？")) -> ()  [unwired: 1 in, 1 out]
      }
    }
  }
  n193 = while "While循环" {
    shift-right: [w437] -> w13
    shift-left: w12 -> [w438]
    tunnel: [w436] -> w8
    tunnel: w11 -> [w434]
    stop <- w432 stop-if-true
    # "HMI命令执行循环（常用）"
    n194 = Dequeue Element(queue=w438, error in (no error)=w434) -> (queue out=w437:refnum<queue>, element=w435:cluster{"命令":string, "数据":variant}, error out=w436:errorcluster)  [unwired: 1 in, 1 out]
    n195 = Unbundle By Name(w435) -> ("命令"=w431:string, "数据"=w433:variant)
    n196 = case shown="\"测试开始\"" w431 {
      tunnel: w433 -> [_ _ _ _ _ _ _ _ _ _ _ _ _]
      tunnel: [_ _ _ _ _ _ _ _ _ _ _ _ w587] -> w432
      frame "空", Default {
      }
      frame "连接" {
        # "设置IP为10. 0.0.100"
        n197 = Current VI's Path() -> (path=w443:path)
        n198 = Strip Path(path=w443) -> (stripped path=w442:path)  [unwired: 1 out]
        n199 = Build Path(base path=w442, name or relative path="Set IP .bat" ("名称或相对路径")) -> (appended path=w445:path)
        n200 = Path To String(path=w445) -> (string=w444:string)
        n201 = call <vilib>:"System Exec.vi"("command line"=w444) -> ("error out"=w441:errorcluster)  [unwired: 7 in, 3 out]
        n202 = call "CreatUTMgrRes.vi"("错误输入（无错误）"=w441) -> ("错误输出"=w440:errorcluster, "返回值"=w439:i32)  [unwired: 9 in]
        n203 = Equal?(x=w439, y=1) -> (x = y?=w447:bool)
        n204 = case shown="真" w447 {
          tunnel: w440 -> [_ _]
          frame False {
            n205 = One Button Dialog(message="连接失败请重试或检查设置！" ("消息")) -> ()  [unwired: 1 in, 1 out]
          }
          frame True {
            w450 = T1."Enabled" ("禁用")
            n206 = property on="采    样" class="Bool (严格)"("DisabledEnum"=w450) -> ()  [unwired: 2 in, 2 out]
            n207 = property on="监    测" class="Bool (严格)"("DisabledEnum"=w450) -> ()  [unwired: 2 in, 2 out]
            n208 = property on="测    试" class="Bool (严格)"("DisabledEnum"=w450) -> ()  [unwired: 2 in, 2 out]
          }
        }
      }
      frame "断开连接" {
        n209 = call "ReleaseUTMgrRes.vi"() -> ("错误输出"=w451:errorcluster)  [unwired: 11 in]
        n210 = To Variant(anything=FALSE) -> (Variant=w453:variant)
        n211 = property on="连接状态" class="Bool"(error in=w451, "Value"=w453) -> ()  [unwired: 1 in, 2 out]
      }
      frame "测量参数设置" {
        n212 = call "测量参数设置.vi"() -> ("错误输出"=w454:errorcluster)  [unwired: 11 in]
        n213 = case shown="无错误" w454 {
          frame No Error {
            n214 = global read "gbl.vi" "声速下限"() -> (w465:dbl)
            n215 = property on="声速下限" class="DigNum (严格)"("Value"=w465) -> (error out=w459:errorcluster)  [unwired: 2 in, 1 out]
            n216 = global read "gbl.vi" "声速上限"() -> (w460:dbl)
            n217 = global read "gbl.vi" "衰减下限"() -> (w464:dbl)
            n218 = property on="声速上限" class="DigNum (严格)"(error in=w459, "Value"=w460) -> (error out=w457:errorcluster)  [unwired: 1 in, 1 out]
            n219 = property on="衰减下限" class="DigNum (严格)"(error in=w457, "Value"=w464) -> (error out=w456:errorcluster)  [unwired: 1 in, 1 out]
            n220 = global read "gbl.vi" "衰减上限"() -> (w458:dbl)
            n221 = global read "gbl.vi" "数据保存路径"() -> (w462:path)
            n222 = property on="衰减上限" class="DigNum (严格)"(error in=w456, "Value"=w458) -> (error out=w455:errorcluster)  [unwired: 1 in, 1 out]
            n223 = global read "gbl.vi" "本次监测名称"() -> (w463:string)
            n224 = property on="本次监测名称" class="Str"(error in=w455, "Value"=w463) -> ()  [unwired: 1 in, 2 out]
            n225 = Path To String(path=w462) -> (string=w461:string)
            n226 = property on="数据导出路径" class="Str"("Value"=w461) -> ()  [unwired: 2 in, 2 out]
          }
          frame Error {
          }
        }
      }
      frame "跳转测量参数设置" {
        # "设置完成打开监测"
        n227 = call "测量参数设置.vi"() -> ("错误输出"=w466:errorcluster)  [unwired: 11 in]
        n228 = case shown="无错误" w466 {
          frame No Error {
            n229 = global read "gbl.vi" "声速下限"() -> (w485:dbl)
            n230 = property on="声速下限" class="DigNum (严格)"("Value"=w485) -> (error out=w481:errorcluster)  [unwired: 2 in, 1 out]
            n231 = global read "gbl.vi" "声速上限"() -> (w482:dbl)
            n232 = global read "gbl.vi" "衰减下限"() -> (w484:dbl)
            n233 = property on="声速上限" class="DigNum (严格)"(error in=w481, "Value"=w482) -> (error out=w479:errorcluster)  [unwired: 1 in, 1 out]
            n234 = property on="采    样" class="Bool (严格)"("DisabledEnum"=T1."Disabled and Grayed Out" ("禁用")) -> ()  [unwired: 2 in, 2 out]
            n235 = property on="衰减下限" class="DigNum (严格)"(error in=w479, "Value"=w484) -> (error out=w478:errorcluster)  [unwired: 1 in, 1 out]
            n236 = global read "gbl.vi" "衰减上限"() -> (w480:dbl)
            n237 = flat-sequence {
              tunnel: [w487] -> w467
              tunnel: w468 -> [w487]
              frame #0 {
                w488 = dbl[] []
                n238 = global write "gbl.vi" "A数组"(w488) -> ()
                n239 = global write "gbl.vi" "V数组"(w488) -> ()
                n240 = global write "gbl.vi" "X数组"(timestamp[] []) -> ()
              }
            }
            n241 = property on="衰减上限" class="DigNum (严格)"(error in=w478, "Value"=w480) -> (error out=w477:errorcluster)  [unwired: 1 in, 1 out]
            n242 = global read "gbl.vi" "本次监测名称"() -> (w483:string)
            n243 = property on="本次监测名称" class="Str"(error in=w477, "Value"=w483) -> (error out=w476:errorcluster)  [unwired: 1 in, 1 out]
            n244 = global read "gbl.vi" "数据保存路径"() -> (w475:path)
            n245 = property on="监测开关" class="Bool (严格)"(error in=w467, "Value"=TRUE) -> ()  [unwired: 1 in, 2 out]
            n246 = Path To String(path=w475) -> (string=w474:string)
            n247 = property on="数据导出路径" class="Str"(error in=w476, "Value"=w474) -> (error out=w472:errorcluster)  [unwired: 1 in, 1 out]
            n248 = property on="实时监测" class="XYGraph (严格)"(error in=w472, "Value"=cluster{"数组":timestamp[], dbl[]}[] [] ("实时监测")) -> (error out=w471:errorcluster)  [unwired: 1 in, 1 out]
            n249 = property on="报警窗" class="MCListbox (严格)"(error in=w471, "ItemNames"=string[][] []) -> (error out=w468:errorcluster)  [unwired: 1 in, 1 out]
          }
          frame Error {
          }
        }
      }
      frame "系统参数设置" {
        n250 = call "系统参数设置.vi"() -> ()  [unwired: 11 in, 1 out]
      }
      frame "测试开始" {
        # "判断是否进行过参数设置"
        n251 = global read "gbl.vi" "声速上限"() -> (w491:dbl)
        n252 = Equal?(x=w491, y=0.0) -> (x = y?=w492:bool)
        n253 = case shown="假" w492 {
          frame False {
            n254 = stacked-sequence {
              frame #0 {
                w501 = dbl[] []
                w500 = dbl[][] []
                # "开始测试时存储全局清空"
                n255 = property on="实时监测" class="XYGraph (严格)"("Value"=cluster{"数组":timestamp[], dbl[]}[] [] ("实时监测")) -> (error out=w497:errorcluster)  [unwired: 2 in, 1 out]
                n256 = property on="报警窗" class="MCListbox (严格)"(error in=w497, "ItemNames"=string[][] []) -> (error out=w494:errorcluster)  [unwired: 1 in, 1 out]
                n257 = global write "gbl.vi" "WaveTime"(w501) -> ()
                n258 = global write "gbl.vi" "WaveData"(w500) -> ()
                n259 = global write "gbl.vi" "计算数据"(w500) -> ()
                n260 = global write "gbl.vi" "A数组"(w501) -> ()
                n261 = global write "gbl.vi" "V数组"(w501) -> ()
                n262 = property on="保存组数" class="DigNum (严格)"(error in=w494, "Value"=0 ("保存组数")) -> (error out=w493:errorcluster)  [unwired: 1 in, 1 out]
                n263 = property on="监测组数" class="DigNum (严格)"(error in=w493, "Value"=0 ("监测组数")) -> ()  [unwired: 1 in, 2 out]
                n264 = global write "gbl.vi" "X数组"(timestamp[] []) -> ()
              }
              frame #1 {
                # "参数全局赋值"
                # "设置游标"
                n265 = global read "gbl.vi" "声速上限"() -> (w510:dbl)
                n266 = global read "gbl.vi" "声速下限"() -> (w511:dbl)
                n267 = global read "gbl.vi" "衰减上限"() -> (w522:dbl)
                n268 = global read "gbl.vi" "衰减下限"() -> (w521:dbl)
                n269 = property on="声速下限" class="DigNum (严格)"("Value"=w511) -> ()  [unwired: 2 in, 2 out]
                n270 = property on="声速上限" class="DigNum (严格)"("Value"=w510) -> ()  [unwired: 2 in, 2 out]
                n271 = property on="衰减下限" class="DigNum (严格)"("Value"=w521) -> ()  [unwired: 2 in, 2 out]
                n272 = property on="衰减上限" class="DigNum (严格)"("Value"=w522) -> ()  [unwired: 2 in, 2 out]
                n273 = global read "gbl.vi" "数据保存路径"() -> (w519:path)
                n274 = global read "gbl.vi" "本次监测名称"() -> (w520:string)
                n275 = formula code="Y1=V1+0.618*(V1-V2);\nY2=V2-0.618*(V1-V2);\nY3=A1+0.618*(A1-A2);\nY4=A2-0.618*(A1-A2);"("V1"=w510, "V2"=w511, "A1"=w522, "A2"=w521) -> ("Y1"=w509:dbl, "Y2"=w508:dbl, "Y3"=w504:dbl, "Y4"=w503:dbl)
                n276 = Path To String(path=w519) -> (string=w518:string)
                n277 = property on="本次监测名称" class="Str"("Value"=w520) -> ()  [unwired: 2 in, 2 out]
                n278 = property on="数据导出路径" class="Str"("Value"=w518) -> ()  [unwired: 2 in, 2 out]
                n279 = property on="实时监测" class="XYGraph (严格)"("ActYScl"=0 ("活动Y标尺"), "YScale.ScaleFit"=u8 0 ("Y标尺.标尺调节"), "YScale.Maximum"=w509, "YScale.Minimum"=w508, "Active Cursor"=u32 0 ("活动游标"), "Cursor.Visible"=TRUE ("游标.可见"), "Cursor.Cursor Y"=w510, "Active Cursor"=u32 1 ("活动游标"), "Cursor.Visible"=TRUE ("游标.可见"), "Cursor.Cursor Y"=w511) -> (error out=w505:errorcluster)  [unwired: 2 in, 1 out]
                n280 = property on="实时监测" class="XYGraph (严格)"(error in=w505, "ActYScl"=1 ("活动Y标尺"), "YScale.ScaleFit"=u8 0 ("Y标尺.标尺调节"), "YScale.Maximum"=w504, "YScale.Minimum"=w503) -> ()  [unwired: 1 in, 2 out]
              }
              frame #2 {
                # "启动测量命令"
                # "测量循环开启"
                n281 = property on="采样开关" class="Bool (严格)"("Value"=FALSE ("采样开关")) -> (error out=w525:errorcluster)  [unwired: 2 in, 1 out]
                n282 = property on="监测开关" class="Bool (严格)"(error in=w525, "Value"=TRUE ("监测开关")) -> (error out=w524:errorcluster)  [unwired: 1 in, 1 out]
                n283 = property on="保存开关" class="Bool (严格)"(error in=w524, "Value"=TRUE ("保存开关")) -> (error out=w523:errorcluster)  [unwired: 1 in, 1 out]
                n284 = Obtain Queue(name (unnamed)="超声测量用" ("名称（未命名）"), element data type=cluster{"命令":string, "数据":variant} {"命令"="", "数据"=variant}, error in (no error)=w523) -> (queue out=w531:refnum<queue>, error out=w530:errorcluster)  [unwired: 2 in, 1 out]
                n285 = Enqueue Element(queue=w531, element=cluster{"命令":string, "数据":variant} {"命令"="测量", "数据"=variant} ("元素"), error in (no error)=w530) -> ()  [unwired: 1 in, 3 out]
              }
            }
          }
          frame True {
            n286 = One Button Dialog(message="请在设置测量参数后再进行测试!" ("消息")) -> (true=w534:bool)  [unwired: 1 in]
            n287 = case shown="真" w534 {
              frame False {
              }
              frame True {
                w538 = T1."Enabled" ("禁用")
                n288 = property on="测    试" class="Bool (严格)"("Value"=FALSE ("测试")) -> (error out=w537:errorcluster)  [unwired: 2 in, 1 out]
                n289 = property on="监    测" class="Bool (严格)"(error in=w537, "DisabledEnum"=w538) -> (error out=w536:errorcluster)  [unwired: 1 in, 1 out]
                n290 = property on="采    样" class="Bool (严格)"(error in=w536, "DisabledEnum"=w538) -> ()  [unwired: 1 in, 2 out]
              }
            }
          }
        }
      }
      frame "关闭测试" {
        w543 = T1."Enabled" ("禁用")
        n291 = property on="采样开关" class="Bool (严格)"("Value"=TRUE) -> (error out=w541:errorcluster)  [unwired: 2 in, 1 out]
        n292 = property on="采    样" class="Bool (严格)"(error in=w541, "DisabledEnum"=w543) -> (error out=w540:errorcluster)  [unwired: 1 in, 1 out]
        n293 = property on="监    测" class="Bool (严格)"(error in=w540, "DisabledEnum"=w543) -> ()  [unwired: 1 in, 2 out]
      }
      frame "导出测试数据" {
        # "关闭测量循环并将全局变量数据导出"
        n294 = property on="数据导出路径" class="Str"() -> ("Value"=w548:string)  [unwired: 2 in, 2 out]
        n295 = property on="报警窗" class="MCListbox (严格)"() -> ("ItemNames"=w546:string[][])  [unwired: 2 in, 2 out]
        n296 = property on="本次监测名称" class="Str"() -> ("Value"=w545:string)  [unwired: 2 in, 2 out]
        n297 = global read "gbl.vi" "计算数据"() -> (w552:dbl[][])
        n298 = String To Path(string=w548) -> (path=w547:path)
        n299 = call "导出监测.vi"("路径"=w547, "报警信息"=w546, "计算数据"=w552, "监测名"=w545) -> ("错误常量 2"=w549:errorcluster)  [unwired: 4 in]
        n300 = global read "gbl.vi" "WaveTime"() -> (w553:dbl[])
        n301 = global read "gbl.vi" "WaveData"() -> (w544:dbl[][])
        n302 = call <vilib>:"Set Busy.vi"("error in (no error)"=w549) -> ("error out"=w551:errorcluster)  [unwired: 9 in, 1 out]
        n303 = call "导出波形.vi"("WaveTime"=w553, "WaveData"=w544, "错误输入"=w551, "保存路径"=w547) -> ("错误输出"=w550:errorcluster)  [unwired: 3 in, 1 out]
        n304 = case shown="无错误" w550 {
          frame No Error {
            n305 = One Button Dialog(message="数据保存成功" ("消息")) -> ()  [unwired: 1 in, 1 out]
          }
          frame Error {
          }
        }
        n306 = call <vilib>:"Unset Busy.vi"("error in (no error)"=w550) -> ()  [unwired: 10 in, 1 out]
      }
      frame "历史数据处理" {
        # "动态调用，并行分支"
        n307 = Current VI's Path() -> (path=w567:path)
        n308 = Strip Path(path=w567) -> (stripped path=w566:path)  [unwired: 1 out]
        n309 = Build Path(base path=w566, name or relative path="子VI\\历史数据.vi" ("名称或相对路径")) -> (appended path=w561:path)
        n310 = Open VI Reference(vi path=w561) -> (vi reference=w562:refnum<vi>, error out=w563:errorcluster)  [unwired: 5 in]
        n311 = invoke class="VI" method="FP.Open"(reference=w562, error in=w563, "Activate"=FALSE ("激活？"), "State"=T3."Standard" ("状态")) -> (reference out=w555:refnum<vi>, error out=w556:errorcluster)  [unwired: 1 in, 3 out]
        n312 = invoke class="VI" method="Run VI"(reference=w555, error in=w556, "Wait until done"=FALSE ("结束前等待"), "Auto Dispose Ref"=TRUE ("自动销毁引用")) -> (reference out=w557:refnum<vi>, error out=w558:errorcluster)  [unwired: 1 in, 3 out]
        n313 = Close Reference(reference=w557, error in (no error)=w558) -> ()  [unwired: 1 out]
      }
      frame "放大实时监测图" {
        n314 = Current VI's Path() -> (path=w570:path)
        n315 = Strip Path(path=w570) -> (stripped path=w571:path)  [unwired: 1 out]
        n316 = Build Path(base path=w571, name or relative path="超声子VI\\实时监测图放大.vi" ("名称或相对路径")) -> (appended path=w576:path)
        n317 = Open VI Reference(vi path=w576) -> (vi reference=w575:refnum<vi>, error out=w574:errorcluster)  [unwired: 5 in]
        n318 = invoke class="VI" method="FP.Open"(reference=w575, error in=w574, "Activate"=FALSE ("激活？"), "State"=T3."Hidden" ("状态")) -> (reference out=w582:refnum<vi>, error out=w581:errorcluster)  [unwired: 1 in, 3 out]
        n319 = invoke class="VI" method="Run VI"(reference=w582, error in=w581, "Wait until done"=FALSE ("结束前等待"), "Auto Dispose Ref"=TRUE ("自动销毁引用")) -> (reference out=w580:refnum<vi>, error out=w579:errorcluster)  [unwired: 1 in, 3 out]
        n320 = Close Reference(reference=w580, error in (no error)=w579) -> ()  [unwired: 1 out]
      }
      frame "前面板消失" {
        n321 = control-ref of="本VI"() -> (w583:refnum<vi>)
        n322 = property class="VI"(reference=w583, "FP:Transparency"=u8 100 ("前面板窗口:透明度")) -> (reference out=w585:refnum<vi>, error out=w586:errorcluster)  [unwired: 1 in]
        n323 = Close Reference(reference=w585, error in (no error)=w586) -> ()  [unwired: 1 out]
      }
      frame "程序停止" {
        n324 = flat-sequence {
          tunnel: [TRUE] -> w587
          frame #0 {
            n325 = control-ref of="本VI"() -> (w590:refnum<vi>)
            n326 = invoke class="VI" method="FP.Close"(reference=w590) -> (reference out=w589:refnum<vi>, error out=w588:errorcluster)  [unwired: 2 in, 1 out]
            n327 = Close Reference(reference=w589, error in (no error)=w588) -> ()  [unwired: 1 out]
          }
          frame #1 {
          }
        }
      }
    }
  }
  n328 = Release Queue(queue=w13, error in (no error)=w8) -> ()  [unwired: 1 in, 3 out]
  n329 = call "ReleaseUTMgrRes.vi"("错误输入（无错误）"=w8) -> ()  [unwired: 10 in, 1 out]
